vi "主界面-内窥缺陷检测.vi"(6 "图片/视频完整路径":path, 7 "图片/视频路径":string, 8 "视频检测帧间隔output":i8, 9 "是否使用GPU计算output":i8, 10 "模式选择output":i8) -> ()   [LabVIEW 2018]
panel:
  out "x+1":i32
  out "输出结果图片路径":path
  out "输出结果文件夹":path caption="路径副本"
  out "Image":T1(plugin-control)
  in  "查看结果图":bool caption="开始检测"
  in  "开始检测":bool
  out "标准输出":string
  out "模式":string
  out "预测结果保存路径":path
  out "预测结果":string
  in  "stop":bool caption="停止"
  out "模型预测进度（请等待）":u8(slide) scale=0.0..180.0
  out "模型所在路径":path
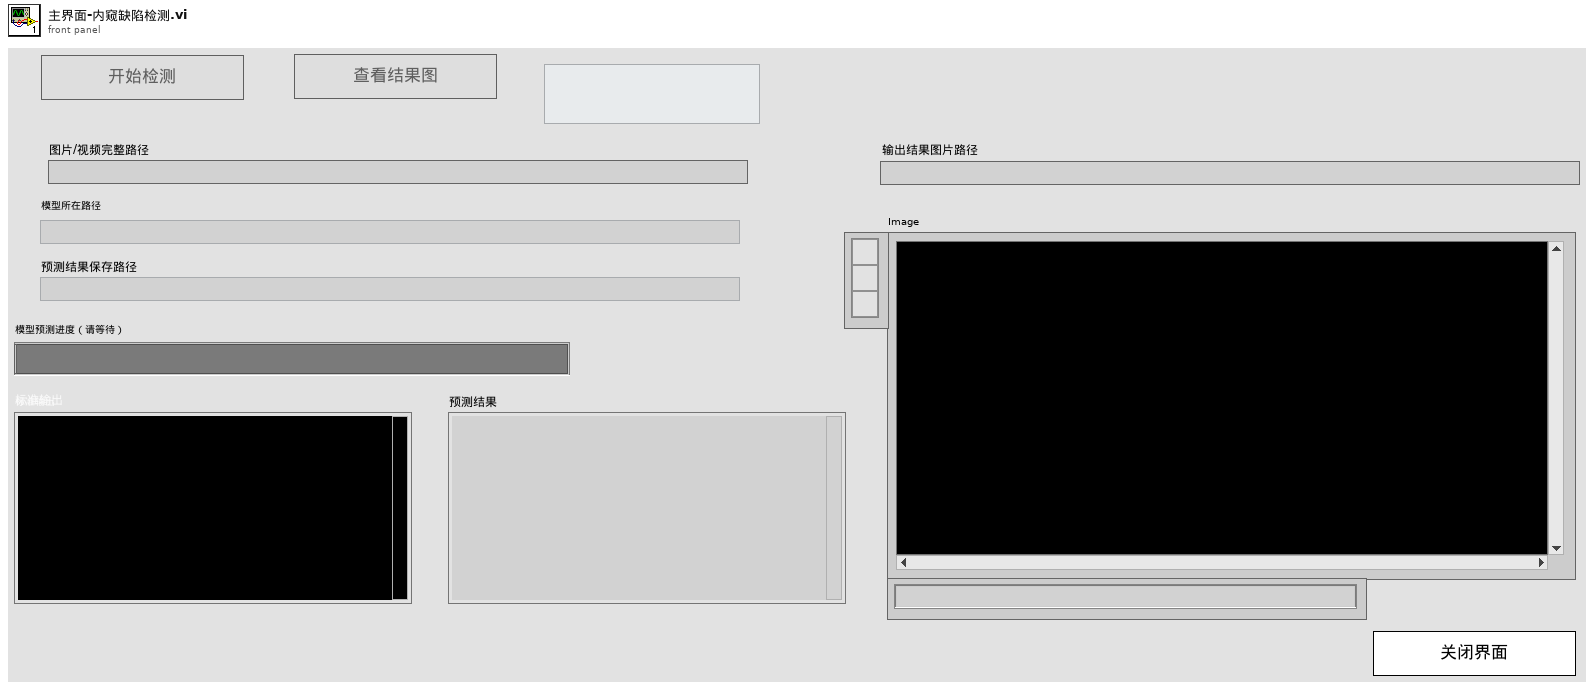
[diagram p1: front panel]
types:
  T1 = typedef "IMAQ Image.ctl" = refnum<image>
  T2 = enum8{"Enabled", "Disabled", "Disabled and Grayed Out"}
  T3 = typedef "Image Type" = u32
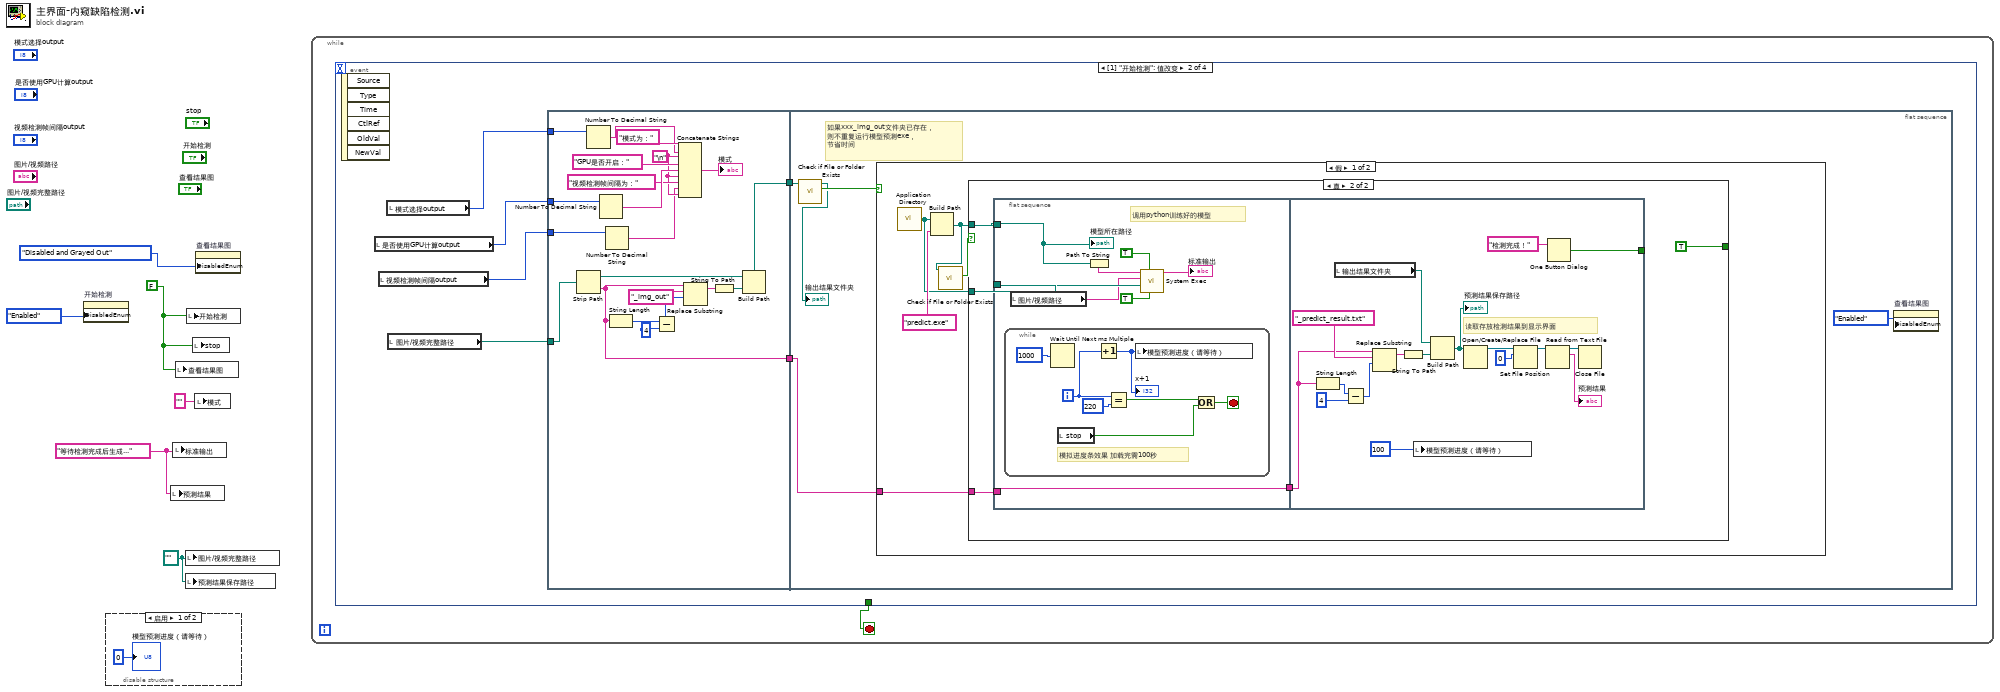
[diagram p0: block diagram]
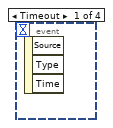
[diagram p3: hidden frame]
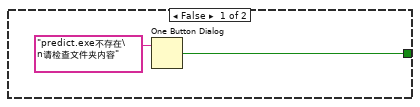
[diagram p4: hidden frame]
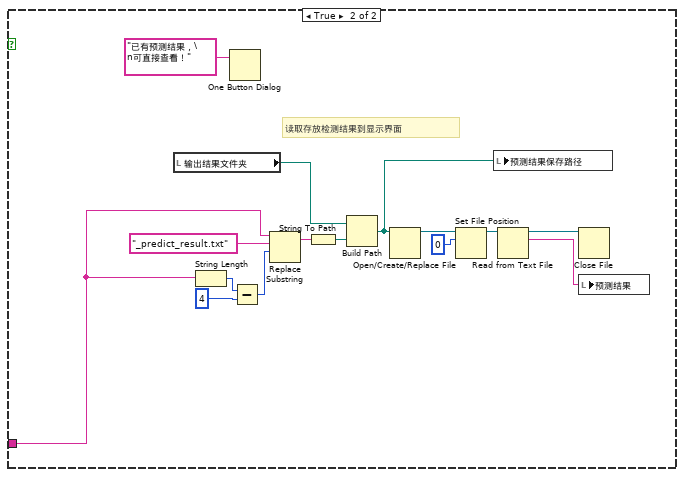
[diagram p5: hidden frame]
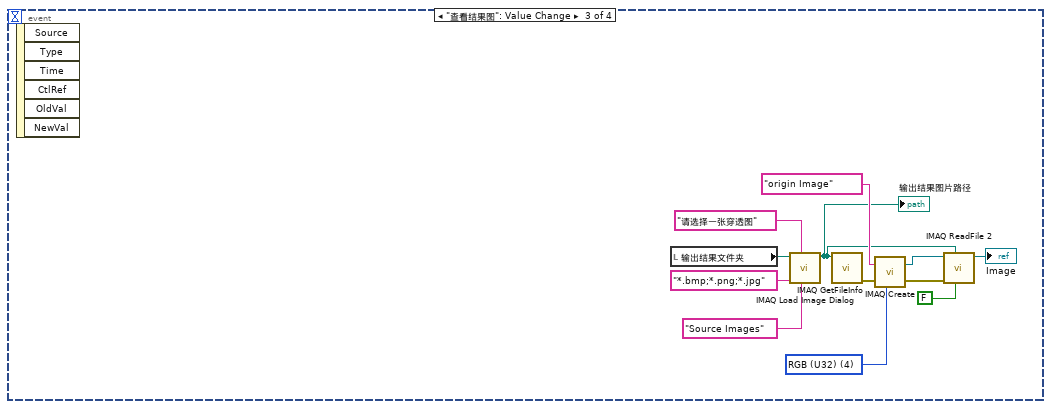
[diagram p6: hidden frame]
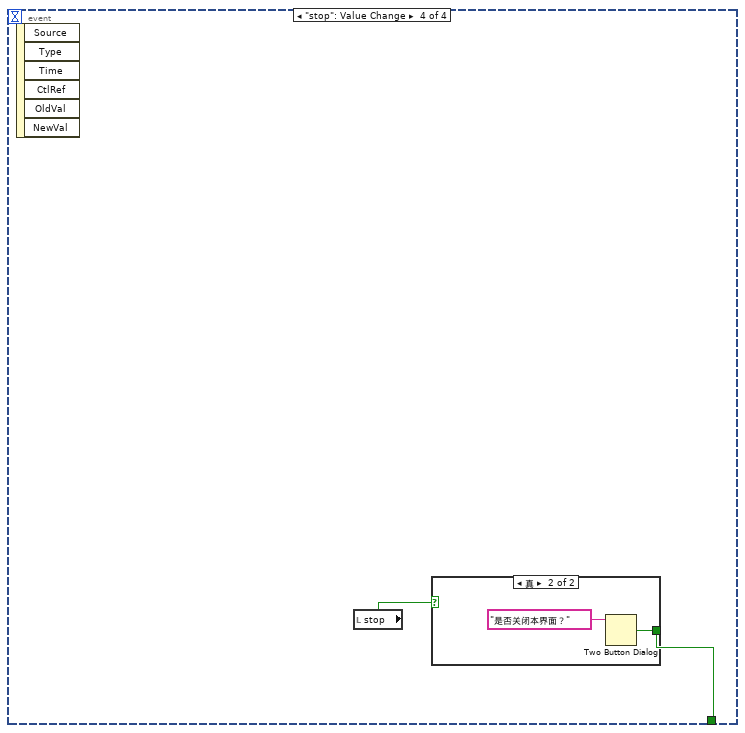
[diagram p7: hidden frame]
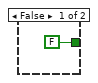
[diagram p8: hidden frame]
diagram:
  w5 = "等待检测完成后生成..."
  w3 = path "" ("图片/视频完整路径")
  w4 = FALSE ("模式选择")
  n1 = property on="开始检测" class="Bool (严格)"("DisabledEnum"=T2."Enabled" ("禁用")) -> ()  [unwired: 2 in, 2 out]
  n2 = disable-structure shown="启用" {
    frame Enabled {
      "模型预测进度（请等待）" <- u8 0 ("模型运行进度")
    }
    frame Disabled {
    }
  }
  n3 = local write "预测结果"(w5) -> ()
  n4 = local write "标准输出"(w5) -> ()
  n5 = local write "查看结果图"(w4) -> ()
  n6 = local write "图片/视频完整路径"(w3) -> ()
  n7 = local write "预测结果保存路径"(w3) -> ()
  n8 = local write "开始检测"(w4) -> ()
  n9 = local write "stop"(w4) -> ()
  n10 = local write "模式"("" ("模式")) -> ()
  n11 = property on="查看结果图" class="Bool (严格)"("DisabledEnum"=T2."Disabled and Grayed Out" ("禁用")) -> ()  [unwired: 2 in, 2 out]
  n12 = while {
    stop <- w8 stop-if-true
    n13 = event shown="[1] \"开始检测\": 值改变" {
      selector: _ -> [_ _ _ _]
      dyn-events: _ -> [_ _ _ _]
      timeout: _ -> [_ _ _ _]
      tunnel: [_ _ _ w112] -> w8
      event Timeout {
        n14 = event-data() -> ()  [unwired: 1 in, 3 out]
      }
      event "开始检测": Value Change {
        n15 = event-data() -> ()  [unwired: 1 in, 6 out]
        n16 = local read "是否使用GPU计算output"() -> (w11:i8)
        n17 = local read "视频检测帧间隔output"() -> (w10:i8)
        n18 = local read "模式选择output"() -> (w12:i8)
        n19 = local read "图片/视频完整路径"() -> (w9:path)
        n20 = flat-sequence {
          tunnel: [w28] -> w14
          tunnel: [w25] -> w13
          tunnel: w12 -> [w15]
          tunnel: w11 -> [w18]
          tunnel: w10 -> [w17]
          tunnel: w9 -> [w16]
          tunnel: w14 -> [w39]
          tunnel: w13 -> [w37]
          frame #0 {
            w20 = "\n"
            n21 = Strip Path(path=w16) -> (stripped path=w35:path, name=w25:string)
            n22 = Number To Decimal String(number=w15) -> (decimal integer string=w23:string)  [unwired: 1 in]
            n23 = Number To Decimal String(number=w18) -> (decimal integer string=w27:string)  [unwired: 1 in]
            n24 = Number To Decimal String(number=w17) -> (decimal integer string=w19:string)  [unwired: 1 in]
            n25 = String Length(string=w25) -> (length=w33:i32)
            n26 = Subtract(x=w33, y=4) -> (x-y=w32:i32)
            n27 = Concatenate Strings("模式为：" ("字符串"), w23, w20, "GPU是否开启：" ("字符串"), w27, w20, "视频检测帧间隔为：" ("字符串"), w19, w20) -> (→"模式":string)
            n28 = Replace Substring(3:w32, 4:"_img_out" ("字符串"), 5:w25) -> (1:w34:string)  [unwired: 1 in, 1 out]
            n29 = String To Path(string=w34) -> (path=w31:path)
            n30 = Build Path(base path=w35, name or relative path=w31) -> (appended path=w28:path)
          }
          frame #1 {
            # "如果xxx_img_out文件夹已存在，\n则不重复运行模型预测exe，\n节省时间"
            n31 = call <vilib>:"Check if File or Folder Exists.vi"("path"=w39) -> ("file or folder exists?"=w40:bool, "dup path"=→"输出结果文件夹":path)  [unwired: 8 in, 1 out]
            n32 = case shown="假" w40 {
              tunnel: w37 -> [w41 w88]
              frame False {
                n33 = call <vilib>:"Application Directory.vi"() -> ("Application Directory"=w43:path)
                n34 = Build Path(base path=w43, name or relative path="predict.exe" ("名称或相对路径")) -> (appended path=w42:path)
                n35 = call <vilib>:"Check if File or Folder Exists.vi"("path"=w42) -> ("file or folder exists?"=w44:bool)  [unwired: 8 in, 2 out]
                n36 = case shown="真" w44 {
                  tunnel: w43 -> [_ w52]
                  tunnel: w42 -> [_ w51]
                  tunnel: [w46 TRUE ("true")] -> _
                  tunnel: w41 -> [_ w48]
                  frame False {
                    n37 = One Button Dialog(message="predict.exe不存在\n请检查文件夹内容" ("消息")) -> (true=w46:bool)  [unwired: 1 in]
                  }
                  frame True {
                    n38 = flat-sequence {
                      tunnel: w52 -> [w56]
                      tunnel: w51 -> [w55]
                      tunnel: [w54] -> w49
                      tunnel: w48 -> [w54]
                      tunnel: w49 -> [w72]
                      tunnel: [w70] -> _
                      frame #0 {
                        # "调用python训练好的模型"
                        n39 = while {
                          i -> [w65]
                          stop <- w61 stop-if-true
                          # "模拟进度条效果 加载完需100秒"
                          n40 = Wait Until Next ms Multiple(millisecond multiple=u32 1000 ("毫秒倍数")) -> ()  [unwired: 1 out]
                          n41 = local read "stop"() -> (w63:bool)
                          n42 = Increment(x=w65) -> (x+1=w66:i32)
                          "x+1" <- w66
                          n43 = Equal?(x=w65, y=220) -> (x = y?=w62:bool)
                          n44 = local write "模型预测进度（请等待）"(w66) -> ()
                          n45 = Or(x=w62, y=w63) -> (x .or. y?=w61:bool)
                        }
                        n46 = local read "图片/视频路径"() -> (w53:string)
                        n47 = Path To String(path=w55) -> (string=w60:string)
                        n48 = call <vilib>:"System Exec.vi"("run minimized? (F)"=TRUE, "wait until completion? (T)"=TRUE, "working directory"=w56, "standard input"=w53, "command line"=w60) -> ("standard output"=→"标准输出":string)  [unwired: 3 in, 3 out]
                        "模型所在路径" <- w55
                      }
                      frame #1 {
                        # "读取存放检测结果到显示界面"
                        n49 = String Length(string=w72) -> (length=w83:i32)
                        n50 = local read "输出结果文件夹"() -> (w69:path)
                        n51 = Subtract(x=w83, y=4) -> (x-y=w84:i32)
                        n52 = Replace Substring(3:w84, 4:"_predict_result.txt" ("字符串"), 5:w72) -> (1:w82:string)  [unwired: 1 in, 1 out]
                        n53 = String To Path(string=w82) -> (path=w81:path)
                        n54 = local write "模型预测进度（请等待）"(u8 100 ("模型预测进度（请等待）")) -> ()
                        n55 = Build Path(base path=w69, name or relative path=w81) -> (appended path=w76:path)
                        "预测结果保存路径" <- w76
                        n56 = Open/Create/Replace File(file path (use dialog)=w76) -> (refnum out=w77:refnum<file>)  [unwired: 5 in, 2 out]
                        n57 = Set File Position(offset (in bytes) (0)=i64 0 ("偏移量（字节）（0）"), refnum=w77) -> (refnum out=w78:refnum<file>)  [unwired: 2 in, 1 out]
                        n58 = Read from Text File(file (use dialog)=w78) -> (refnum out=w80:refnum<file>, text=→"预测结果":string)  [unwired: 3 in, 2 out]
                        n59 = One Button Dialog(message="检测完成！" ("消息")) -> (true=w70:bool)  [unwired: 1 in]
                        n60 = Close File(refnum=w80) -> ()  [unwired: 1 in, 2 out]
                      }
                    }
                  }
                }
              }
              frame True {
                # "读取存放检测结果到显示界面"
                n61 = local read "输出结果文件夹"() -> (w85:path)
                n62 = String Length(string=w88) -> (length=w90:i32)
                n63 = One Button Dialog(message="已有预测结果，\n可直接查看！" ("消息")) -> ()  [unwired: 1 in, 1 out]
                n64 = Subtract(x=w90, y=4) -> (x-y=w89:i32)
                n65 = Replace Substring(3:w89, 4:"_predict_result.txt" ("字符串"), 5:w88) -> (1:w91:string)  [unwired: 1 in, 1 out]
                n66 = String To Path(string=w91) -> (path=w92:path)
                n67 = Build Path(base path=w85, name or relative path=w92) -> (appended path=w87:path)
                n68 = Open/Create/Replace File(file path (use dialog)=w87) -> (refnum out=w95:refnum<file>)  [unwired: 5 in, 2 out]
                n69 = Set File Position(offset (in bytes) (0)=i64 0 ("偏移量（字节）（0）"), refnum=w95) -> (refnum out=w94:refnum<file>)  [unwired: 2 in, 1 out]
                n70 = local write "预测结果保存路径"(w87) -> ()
                n71 = Read from Text File(file (use dialog)=w94) -> (refnum out=w93:refnum<file>, text=w86:string)  [unwired: 3 in, 2 out]
                n72 = Close File(refnum=w93) -> ()  [unwired: 1 in, 2 out]
                n73 = local write "预测结果"(w86) -> ()
              }
            }
            n74 = property on="查看结果图" class="Bool (严格)"("DisabledEnum"=T2."Enabled" ("禁用")) -> ()  [unwired: 2 in, 2 out]
          }
        }
      }
      event "查看结果图": Value Change {
        w107 = T3 4 items=["Grayscale (U8)", "Grayscale (I16)", "Grayscale (SGL)", "Complex (CSG)", "RGB (U32)", "HSL (U32)", "RGB (U64)", "Grayscale (U16)"] ("Image Type")
        n75 = event-data() -> ()  [unwired: 1 in, 6 out]
        n76 = local read "输出结果文件夹"() -> (w101:path)
        n77 = call "IMAQ Load Image Dialog"("Pattern Label"="Source Images", "Prompt"="请选择一张穿透图" ("prompt"), "Pattern"="*.bmp;*.png;*.jpg", "Start Path"=w101) -> ("Path"=w100:path)  [unwired: 5 in, 2 out]
        "输出结果图片路径" <- w100
        n78 = call "IMAQ GetFileInfo"("File Path"=w100) -> ("error out"=w109:errorcluster)  [unwired: 4 in, 6 out]
        n79 = call "IMAQ Create"("Image Name"="origin Image", "Image Type"=w107, "error in (no error)"=w109) -> ("New Image"=w110:T1, "error out"=w111:errorcluster)  [unwired: 2 in]
        n80 = call "IMAQ ReadFile 2"("Use File Path Image Type"=FALSE, "File Path"=w100, "error in (no error)"=w111, "Image"=w110) -> ("Image Out"=→"Image":T1)  [unwired: 3 in, 4 out]
      }
      event "stop": Value Change {
        n81 = event-data() -> ()  [unwired: 1 in, 6 out]
        n82 = local read "stop"() -> (w113:bool)
        n83 = case shown="真" w113 {
          tunnel: [FALSE ("T button?") w115] -> w112
          frame False {
          }
          frame True {
            n84 = Two Button Dialog(message="是否关闭本界面？" ("消息")) -> (T button?=w115:bool)  [unwired: 2 in]
          }
        }
      }
    }
  }
